vi "DoubleToSetpoint.vi"(1 "Double":dbl) -> (0 "SP":u8[](array[numeric]))   [LabVIEW 2021]
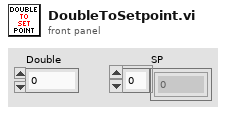
[diagram p1: front panel]
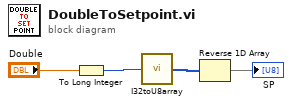
[diagram p0: block diagram]
diagram:
  n1 = To Long Integer(number="Double") -> (32bit integer=w3:i32)
  n2 = call "I32toU8array.vi"("I32"=w3) -> ("U8"=w4:u8[])
  n3 = Reverse 1D Array(array=w4) -> (reversed array=→"SP":u8[])
